vi "HFRR ADV v05 new software.vi"() -> ()   [LabVIEW 2025] (continued)
              tunnel: [w2074] -> w1919 mode=indexing
              tunnel: [w2070] -> w1894 mode=indexing
              tunnel: [w2066] -> w1875 mode=indexing
              tunnel: [w2061] -> w1833 mode=indexing
              (unwired) TRUE ("line mode (F)")
              n1812 = Read from Text File "Read File"(file (use dialog)=w2097, error in=w2096) -> (text=w2062:string)  [unwired: 2 in, 3 out]
              n1813 = local write "String 7"(w2062) -> ()
              n1814 = String Subset(string=w2062, offset (0)=85, length (rest)=9 ("length (rest)")) -> (substring=w2065:string)
              n1815 = String Subset(string=w2062, offset (0)=35, length (rest)=9 ("length (rest)")) -> (substring=w2087:string)
              n1816 = String Subset(string=w2062, offset (0)=55, length (rest)=9 ("length (rest)")) -> (substring=w2073:string)
              n1817 = String Subset(string=w2062, offset (0)=25, length (rest)=9 ("length (rest)")) -> (substring=w2067:string)
              n1818 = String Subset(string=w2062, offset (0)=45, length (rest)=9 ("length (rest)")) -> (substring=w2075:string)
              n1819 = String Subset(string=w2062, offset (0)=0, length (rest)=14 ("length (rest)")) -> (substring=w2090:string)
              n1820 = String Subset(string=w2062, offset (0)=15, length (rest)=9 ("length (rest)")) -> (substring=w2093:string)
              n1821 = String Subset(string=w2062, offset (0)=65, length (rest)=9 ("length (rest)")) -> (substring=w2079:string)
              n1822 = Fract/Exp String To Number(string=w2065) -> (number=w2061:dbl)  [unwired: 3 in, 1 out]
              n1823 = Fract/Exp String To Number(string=w2087) -> (number=w2085:dbl)  [unwired: 3 in, 1 out]
              n1824 = Fract/Exp String To Number(string=w2073) -> (number=w2070:dbl)  [unwired: 3 in, 1 out]
              n1825 = Fract/Exp String To Number(string=w2067) -> (number=w2066:dbl)  [unwired: 3 in, 1 out]
              n1826 = Fract/Exp String To Number(string=w2075) -> (number=w2074:dbl)  [unwired: 3 in, 1 out]
              n1827 = Fract/Exp String To Number(string=w2090) -> (number=w2086:dbl)  [unwired: 3 in, 1 out]
              n1828 = Fract/Exp String To Number(string=w2093) -> (number=w2084:dbl)  [unwired: 3 in, 1 out]
              n1829 = Fract/Exp String To Number(string=w2079) -> (number=w2082:dbl)  [unwired: 3 in, 1 out]
              n1830 = Add(x=w2082, y=0.0) -> (x+y=w2078:dbl)
            }
            n1831 = for {
              N: w1970 -> [_]
              tunnel: w1977 -> [w2025]
              tunnel: w1976 -> [w2024]
              tunnel: [w2014] -> w1930 mode=indexing
              tunnel: [w2013] -> w1923 mode=indexing
              tunnel: w1967 -> [_]
              tunnel: [w2002] -> w1928 mode=indexing
              tunnel: [w2007] -> w1925 mode=indexing
              tunnel: [w2003] -> w1915 mode=indexing
              tunnel: [w1998] -> w1890 mode=indexing
              tunnel: [w1994] -> w1871 mode=indexing
              tunnel: [w1989] -> w1831 mode=indexing
              (unwired) 1.0 ("x")
              (unwired) TRUE ("line mode (F)")
              n1832 = Read from Text File "Read File"(file (use dialog)=w2025, error in=w2024) -> (text=w1990:string)  [unwired: 2 in, 3 out]
              n1833 = local write "String 12"(w1990) -> ()
              n1834 = String Subset(string=w1990, offset (0)=85, length (rest)=9 ("length (rest)")) -> (substring=w1992:string)
              n1835 = String Subset(string=w1990, offset (0)=35, length (rest)=9 ("length (rest)")) -> (substring=w2015:string)
              n1836 = String Subset(string=w1990, offset (0)=55, length (rest)=9 ("length (rest)")) -> (substring=w2000:string)
              n1837 = String Subset(string=w1990, offset (0)=25, length (rest)=9 ("length (rest)")) -> (substring=w1996:string)
              n1838 = String Subset(string=w1990, offset (0)=45, length (rest)=9 ("length (rest)")) -> (substring=w2005:string)
              n1839 = String Subset(string=w1990, offset (0)=15, length (rest)=9 ("length (rest)")) -> (substring=w2021:string)
              n1840 = String Subset(string=w1990, offset (0)=0, length (rest)=14 ("length (rest)")) -> (substring=w2018:string)
              n1841 = String Subset(string=w1990, offset (0)=65, length (rest)=9 ("length (rest)")) -> (substring=w2008:string)
              n1842 = Fract/Exp String To Number(string=w1992) -> (number=w1989:dbl)  [unwired: 3 in, 1 out]
              n1843 = Fract/Exp String To Number(string=w2015) -> (number=w2013:dbl)  [unwired: 3 in, 1 out]
              n1844 = Fract/Exp String To Number(string=w2000) -> (number=w1998:dbl)  [unwired: 3 in, 1 out]
              n1845 = Fract/Exp String To Number(string=w1996) -> (number=w1994:dbl)  [unwired: 3 in, 1 out]
              n1846 = Fract/Exp String To Number(string=w2005) -> (number=w2003:dbl)  [unwired: 3 in, 1 out]
              n1847 = Fract/Exp String To Number(string=w2021) -> (number=w2002:dbl)  [unwired: 3 in, 1 out]
              n1848 = Fract/Exp String To Number(string=w2018) -> (number=w2014:dbl)  [unwired: 3 in, 1 out]
              n1849 = Fract/Exp String To Number(string=w2008) -> (number=w2011:dbl)  [unwired: 3 in, 1 out]
              n1850 = Add(x=w2011, y=0.0) -> (x+y=w2007:dbl)
            }
            n1851 = Delete From Array(array=w1873, index=0) -> (array with subset deleted=w1846:dbl[])  [unwired: 1 in, 1 out]
            n1852 = Delete From Array(array=w1936, index=0) -> (array with subset deleted=w1909:dbl[])  [unwired: 1 in, 1 out]
            n1853 = Delete From Array(array=w1916, index=0) -> (array with subset deleted=w1904:dbl[])  [unwired: 1 in, 1 out]
            n1854 = Delete From Array(array=w1934, index=0) -> (array with subset deleted=w1935:dbl[])  [unwired: 1 in, 1 out]
            n1855 = call-poly <vilib>:"Mean.vi"("X"=w1846) -> ("mean"=→"КОФ2 4":dbl)  [unwired: 1 out]
            n1856 = call-poly <vilib>:"Mean.vi"("X"=w1909) -> ("mean"=→"КОФ3":dbl)  [unwired: 1 out]
            n1857 = call-poly <vilib>:"Mean.vi"("X"=w1904) -> ("mean"=→"CP3":dbl)  [unwired: 1 out]
            n1858 = Delete From Array(array=w1898, index=0) -> (array with subset deleted=w1825:dbl[])  [unwired: 1 in, 1 out]
            n1859 = Delete From Array(array=w1837, index=0) -> (array with subset deleted=w1824:dbl[])  [unwired: 1 in, 1 out]
            n1860 = Delete From Array(array=w1877, index=0) -> (array with subset deleted=w1848:dbl[])  [unwired: 1 in, 1 out]
            n1861 = Delete From Array(array=w1955, index=0) -> (array with subset deleted=w1910:dbl[])  [unwired: 1 in, 1 out]
            n1862 = Delete From Array(array=w1921, index=0) -> (array with subset deleted=w1906:dbl[])  [unwired: 1 in, 1 out]
            "array w/ subset deleted" <- w1906
            n1863 = Delete From Array(array=w1952, index=0) -> (array with subset deleted=w1953:dbl[])  [unwired: 1 in, 1 out]
            n1864 = call-poly <vilib>:"Mean.vi"("X"=w1848) -> ("mean"=→"КОФ2 2":dbl)  [unwired: 1 out]
            n1865 = call-poly <vilib>:"Mean.vi"("X"=w1910) -> ("mean"=→"КОФ1":dbl)  [unwired: 1 out]
            n1866 = Bundle "Bundle"(w1825, w1824) -> (w1830:cluster{dbl[], dbl[]})  [unwired: 1 in]
            n1867 = Bundle "Bundle"(w1825, w1953) -> (w1817:cluster{dbl[], dbl[]})  [unwired: 1 in]
            n1868 = Delete From Array(array=w1832, index=0) -> (array with subset deleted=w1820:dbl[])  [unwired: 1 in, 1 out]
            n1869 = Delete From Array(array=w1833, index=0) -> (array with subset deleted=w1822:dbl[])  [unwired: 1 in, 1 out]
            n1870 = Delete From Array(array=w1943, index=0) -> (array with subset deleted=w1944:dbl[])  [unwired: 1 in, 1 out]
            n1871 = Delete From Array(array=w1831, index=0) -> (array with subset deleted=w1818:dbl[])  [unwired: 1 in, 1 out]
            n1872 = Delete From Array(array=w1925, index=0) -> (array with subset deleted=w1926:dbl[])  [unwired: 1 in, 1 out]
            n1873 = Delete From Array(array=w1950, index=0) -> (array with subset deleted=w1856:dbl[])  [unwired: 1 in, 1 out]
            n1874 = Delete From Array(array=w1896, index=0) -> (array with subset deleted=w1852:dbl[])  [unwired: 1 in, 1 out]
            n1875 = Delete From Array(array=w1932, index=0) -> (array with subset deleted=w1854:dbl[])  [unwired: 1 in, 1 out]
            n1876 = Delete From Array(array=w1892, index=0) -> (array with subset deleted=w1850:dbl[])  [unwired: 1 in, 1 out]
            n1877 = Delete From Array(array=w1941, index=0) -> (array with subset deleted=w1855:dbl[])  [unwired: 1 in, 1 out]
            n1878 = Delete From Array(array=w1894, index=0) -> (array with subset deleted=w1851:dbl[])  [unwired: 1 in, 1 out]
            n1879 = Delete From Array(array=w1875, index=0) -> (array with subset deleted=w1847:dbl[])  [unwired: 1 in, 1 out]
            n1880 = Delete From Array(array=w1919, index=0) -> (array with subset deleted=w1905:dbl[])  [unwired: 1 in, 1 out]
            n1881 = Delete From Array(array=w1946, index=0) -> (array with subset deleted=w1907:dbl[])  [unwired: 1 in, 1 out]
            n1882 = Delete From Array(array=w1923, index=0) -> (array with subset deleted=w1853:dbl[])  [unwired: 1 in, 1 out]
            n1883 = Delete From Array(array=w1890, index=0) -> (array with subset deleted=w1849:dbl[])  [unwired: 1 in, 1 out]
            n1884 = Delete From Array(array=w1871, index=0) -> (array with subset deleted=w1845:dbl[])  [unwired: 1 in, 1 out]
            n1885 = Delete From Array(array=w1915, index=0) -> (array with subset deleted=w1903:dbl[])  [unwired: 1 in, 1 out]
            n1886 = Delete From Array(array=w1928, index=0) -> (array with subset deleted=w1908:dbl[])  [unwired: 1 in, 1 out]
            n1887 = Delete From Array(array=w1938, index=0) -> (array with subset deleted=w1821:dbl[])  [unwired: 1 in, 1 out]
            n1888 = Delete From Array(array=w1948, index=0) -> (array with subset deleted=w1823:dbl[])  [unwired: 1 in, 1 out]
            n1889 = Delete From Array(array=w1930, index=0) -> (array with subset deleted=w1819:dbl[])  [unwired: 1 in, 1 out]
            n1890 = Bundle "Bundle"(w1825, w1856) -> (w1843:cluster{dbl[], dbl[]})  [unwired: 1 in]
            n1891 = Bundle "Bundle"(w1825, w1910) -> (w1844:cluster{dbl[], dbl[]})  [unwired: 1 in]
            n1892 = Bundle "Bundle"(w1856, w1852) -> (w1858:cluster{dbl[], dbl[]})  [unwired: 1 in]
            n1893 = Bundle "Bundle"(w1821, w1820) -> (w1828:cluster{dbl[], dbl[]})  [unwired: 1 in]
            n1894 = Bundle "Bundle"(w1854, w1850) -> (w1860:cluster{dbl[], dbl[]})  [unwired: 1 in]
            n1895 = Bundle "Bundle"(w1821, w1854) -> (w1964:cluster{dbl[], dbl[]})  [unwired: 1 in]
            n1896 = Bundle "Bundle"(w1821, w1850) -> (w1888:cluster{dbl[], dbl[]})  [unwired: 1 in]
            n1897 = Bundle "Bundle"(w1821, w1909) -> (w1974:cluster{dbl[], dbl[]})  [unwired: 1 in]
            n1898 = Bundle "Bundle"(w1821, w1904) -> (w1912:cluster{dbl[], dbl[]})  [unwired: 1 in]
            n1899 = Bundle "Bundle"(w1821, w1935) -> (w1959:cluster{dbl[], dbl[]})  [unwired: 1 in]
            n1900 = Bundle "Bundle"(w1855, w1851) -> (w1859:cluster{dbl[], dbl[]})  [unwired: 1 in]
            n1901 = Bundle "Bundle"(w1823, w1822) -> (w1829:cluster{dbl[], dbl[]})  [unwired: 1 in]
            n1902 = Bundle "Bundle"(w1823, w1855) -> (w1966:cluster{dbl[], dbl[]})  [unwired: 1 in]
            n1903 = Bundle "Bundle"(w1823, w1851) -> (w1889:cluster{dbl[], dbl[]})  [unwired: 1 in]
            n1904 = Bundle "Bundle"(w1823, w1905) -> (w1913:cluster{dbl[], dbl[]})  [unwired: 1 in]
            n1905 = Bundle "Bundle"(w1823, w1907) -> (w1975:cluster{dbl[], dbl[]})  [unwired: 1 in]
            n1906 = Bundle "Bundle"(w1823, w1944) -> (w1957:cluster{dbl[], dbl[]})  [unwired: 1 in]
            n1907 = Bundle "Bundle"(w1853, w1849) -> (w1861:cluster{dbl[], dbl[]})  [unwired: 1 in]
            n1908 = Bundle "Bundle"(w1819, w1818) -> (w1827:cluster{dbl[], dbl[]})  [unwired: 1 in]
            n1909 = Bundle "Bundle"(w1819, w1853) -> (w1965:cluster{dbl[], dbl[]})  [unwired: 1 in]
            n1910 = Bundle "Bundle"(w1819, w1849) -> (w1887:cluster{dbl[], dbl[]})  [unwired: 1 in]
            n1911 = Bundle "Bundle"(w1819, w1903) -> (w1911:cluster{dbl[], dbl[]})  [unwired: 1 in]
            n1912 = Bundle "Bundle"(w1819, w1908) -> (w1973:cluster{dbl[], dbl[]})  [unwired: 1 in]
            n1913 = Bundle "Bundle"(w1819, w1926) -> (w1958:cluster{dbl[], dbl[]})  [unwired: 1 in]
            n1914 = call-poly <vilib>:"Mean.vi"("X"=w1906) -> ("mean"=→"CP1":dbl)  [unwired: 1 out]
            n1915 = call-poly <vilib>:"Mean.vi"("X"=w1847) -> ("mean"=→"КОФ2 3":dbl)  [unwired: 1 out]
            n1916 = call-poly <vilib>:"Mean.vi"("X"=w1905) -> ("mean"=→"CP2":dbl)  [unwired: 1 out]
            n1917 = call-poly <vilib>:"Mean.vi"("X"=w1907) -> ("mean"=→"КОФ2":dbl)  [unwired: 1 out]
            n1918 = call-poly <vilib>:"Mean.vi"("X"=w1845) -> ("mean"=→"КОФ2 5":dbl)  [unwired: 1 out]
            n1919 = call-poly <vilib>:"Mean.vi"("X"=w1903) -> ("mean"=→"CP4":dbl)  [unwired: 1 out]
            n1920 = call-poly <vilib>:"Mean.vi"("X"=w1908) -> ("mean"=→"КОФ4":dbl)  [unwired: 1 out]
            n1921 = Bundle "Bundle"(w1825, w1852) -> (w1816:cluster{dbl[], dbl[]})  [unwired: 1 in]
            n1922 = Bundle "Bundle"(w1825, w1906) -> (w1839:cluster{dbl[], dbl[]})  [unwired: 1 in]
            n1923 = Build Array "Build Array"(w1816, w1839) -> (w1842:cluster{dbl[], dbl[]}[])
            "XY Graph 17" <- w1842
            n1924 = Build Array "Build Array"(w1830, w1829, w1828, w1827) -> (→"Frequency ( Hz )":cluster{dbl[], dbl[]}[])
            n1925 = Build Array "Build Array"(w1858, w1859, w1860, w1861) -> (→"Air Temp ( °C ) vs Humidity ( % RH )":cluster{dbl[], dbl[]}[])
            n1926 = Build Array "Build Array"(w1843, w1966, w1964, w1965) -> (→"Air Temperature  ( °C )":cluster{dbl[], dbl[]}[])
            n1927 = Build Array "Build Array"(w1816, w1889, w1888, w1887) -> (→"Humidity ( %RH )":cluster{dbl[], dbl[]}[])
            n1928 = Build Array "Build Array"(w1844, w1975, w1974, w1973) -> (→"Coefficient Of Friction":cluster{dbl[], dbl[]}[])
            n1929 = Build Array "Build Array"(w1839, w1913, w1912, w1911) -> (→"Sample Temperature ( °C )":cluster{dbl[], dbl[]}[])
            n1930 = Build Array "Build Array"(w1817, w1957, w1959, w1958) -> (→"XY Graph 13":cluster{dbl[], dbl[]}[])
            n1931 = Bundle "Bundle"(w1825, w1848) -> (w1870:cluster{dbl[], dbl[]})  [unwired: 1 in]
            n1932 = Bundle "Bundle"(w1821, w1846) -> (w1868:cluster{dbl[], dbl[]})  [unwired: 1 in]
            n1933 = Bundle "Bundle"(w1823, w1847) -> (w1869:cluster{dbl[], dbl[]})  [unwired: 1 in]
            n1934 = Bundle "Bundle"(w1819, w1845) -> (w1867:cluster{dbl[], dbl[]})  [unwired: 1 in]
            n1935 = Build Array "Build Array"(w1870, w1869, w1868, w1867) -> (→"Stroke ( mm )":cluster{dbl[], dbl[]}[])
            n1936 = local write "XY Graph 16"(w1842) -> ()
          }
          frame #2 {
          }
          frame #3 {
            n1937 = local write "Numeric 8"(0 ("Numeric 8")) -> ()
            n1938 = local write "Numeric 11"(0 ("Numeric 11")) -> ()
            n1939 = local write "Numeric 12"(0 ("Numeric 12")) -> ()
            n1940 = local write "Numeric 13"(0 ("Numeric 13")) -> ()
            n1941 = property on="OPEN" class="Bool (strict)"("Visible"=TRUE) -> ()  [unwired: 2 in, 2 out]
            n1942 = local read "String Control 2"() -> (w2142:string)
            n1943 = local read "String Control 4"() -> (w2141:string)
            n1944 = local read "String Control 6"() -> (w2140:string)
            n1945 = local read "String Control 8"() -> (w2139:string)
            n1946 = Match Pattern(string=w2142, regular expression="Samples / cycle :- ") -> (after substring=w2156:string)  [unwired: 1 in, 3 out]
            n1947 = Match Pattern(string=w2142, regular expression="Frequency :- ") -> (after substring=w2175:string)  [unwired: 1 in, 3 out]
            n1948 = Match Pattern(string=w2141, regular expression="Samples / cycle :- ") -> (after substring=w2152:string)  [unwired: 1 in, 3 out]
            n1949 = Match Pattern(string=w2141, regular expression="Frequency :- ") -> (after substring=w2170:string)  [unwired: 1 in, 3 out]
            n1950 = Match Pattern(string=w2140, regular expression="Samples / cycle :- ") -> (after substring=w2148:string)  [unwired: 1 in, 3 out]
            n1951 = Match Pattern(string=w2140, regular expression="Frequency :- ") -> (after substring=w2165:string)  [unwired: 1 in, 3 out]
            n1952 = Match Pattern(string=w2139, regular expression="Samples / cycle :- ") -> (after substring=w2144:string)  [unwired: 1 in, 3 out]
            n1953 = Match Pattern(string=w2139, regular expression="Frequency :- ") -> (after substring=w2160:string)  [unwired: 1 in, 3 out]
            n1954 = String Subset(string=w2156, length (rest)=6 ("length (rest)")) -> (substring=w2158:string)  [unwired: 1 in]
            n1955 = String Subset(string=w2175, length (rest)=9 ("length (rest)")) -> (substring=w2177:string)  [unwired: 1 in]
            n1956 = String Subset(string=w2152, length (rest)=6 ("length (rest)")) -> (substring=w2154:string)  [unwired: 1 in]
            n1957 = String Subset(string=w2170, length (rest)=9 ("length (rest)")) -> (substring=w2172:string)  [unwired: 1 in]
            n1958 = String Subset(string=w2148, length (rest)=6 ("length (rest)")) -> (substring=w2150:string)  [unwired: 1 in]
            n1959 = String Subset(string=w2165, length (rest)=9 ("length (rest)")) -> (substring=w2167:string)  [unwired: 1 in]
            n1960 = String Subset(string=w2144, length (rest)=6 ("length (rest)")) -> (substring=w2146:string)  [unwired: 1 in]
            n1961 = String Subset(string=w2160, length (rest)=9 ("length (rest)")) -> (substring=w2162:string)  [unwired: 1 in]
            n1962 = Fract/Exp String To Number(string=w2158) -> (number=w2138:dbl)  [unwired: 3 in, 1 out]
            n1963 = Fract/Exp String To Number(string=w2177) -> (number=w2178:dbl)  [unwired: 3 in, 1 out]
            n1964 = Fract/Exp String To Number(string=w2154) -> (number=w2137:dbl)  [unwired: 3 in, 1 out]
            n1965 = Fract/Exp String To Number(string=w2172) -> (number=w2173:dbl)  [unwired: 3 in, 1 out]
            n1966 = Fract/Exp String To Number(string=w2150) -> (number=w2136:dbl)  [unwired: 3 in, 1 out]
            n1967 = Fract/Exp String To Number(string=w2167) -> (number=w2168:dbl)  [unwired: 3 in, 1 out]
            n1968 = Fract/Exp String To Number(string=w2146) -> (number=w2135:dbl)  [unwired: 3 in, 1 out]
            n1969 = Fract/Exp String To Number(string=w2162) -> (number=w2163:dbl)  [unwired: 3 in, 1 out]
            n1970 = local write "sample1"(w2138) -> ()
            n1971 = local write "freq1"(w2178) -> ()
            n1972 = local write "sample2"(w2137) -> ()
            n1973 = local write "freq2"(w2173) -> ()
            n1974 = local write "sample3"(w2136) -> ()
            n1975 = local write "freq3"(w2168) -> ()
            n1976 = local write "sample4"(w2135) -> ()
            n1977 = local write "freq 4"(w2163) -> ()
          }
        }
      }
    }
    n1978 = case shown="True" w1627 {
      selector: w1627 -> [_ w1755]
      frame False {
      }
      frame True {
        n1979 = Not(x=w1755) -> (.not. x?=w1751:bool)
        n1980 = local write "service 3"(w1751) -> ()
        n1981 = local write "OPEN 6"(w1751) -> ()
        n1982 = call <vilib>:"System Exec.vi"("wait until completion? (T)"=TRUE, "command line"="C:\\LAB-IQ\\Scar View.exe") -> ("error out"=→"error out 5":errorcluster)  [unwired: 6 in, 3 out]
      }
    }
    n1983 = case shown="\"Acquire\", Default" w1638 {
      frame "Acquire", Default {
        w2651 = 0.2 ("y")
        w2656 = 1.0 ("y")
        w2657 = 0.8 ("y")
        # "Elapsed time\ncof\nstroke\nAir temp\nTemp\nHumidity"
        n1984 = disable-structure shown="Disabled" {
          frame Disabled {
            n1985 = local read "Flag"() -> (w2674:dbl)
            n1986 = local read "RUN"() -> (w2671:bool)
            n1987 = Not(x=w2671) -> (.not. x?=w2670:bool)
            n1988 = Equal?(x=w2674, y=10.0) -> (x = y?=w2672:bool)
            n1989 = And(x=w2672, y=w2670) -> (x .and. y?=w2669:bool)
            n1990 = case shown="True" w2669 {
              frame False {
              }
              frame True {
                w2675 = FALSE ("Heater Button")
                n1991 = local write "Humidity"(w2675) -> ()
                n1992 = local write "Heater Button"(w2675) -> ()
              }
            }
          }
          frame Enabled {
          }
        }
        n1993 = disable-structure shown="Disabled" {
          frame Disabled {
            n1994 = case shown="True" {
              selector: _ -> [_ _]
              frame False {
              }
              frame True {
                w2766 = TRUE ("Heater")
                n1995 = local write "Humidity"(w2766) -> ()
                n1996 = local write "Heater Button"(w2766) -> ()
                n1997 = local read "TEST STANDARD"() -> (w2769:T3)
                n1998 = local read "TEST STANDARD"() -> (w2764:T3)
                n1999 = Equal?(x=w2769, y=enum16{"ASTM D6079", "ISO 12156", "Custom"}."ISO 12156" ("Test Standard")) -> (x = y?=w2767:bool)
                n2000 = Equal?(x=w2764, y=enum16{"ASTM D6079", "ISO 12156", "Custom"}."ASTM D6079" ("Test Standard")) -> (x = y?=w2763:bool)
                n2001 = case shown="True" w2767 {
                  frame False {
                  }
                  frame True {
                    n2002 = local write "Heater"(TRUE ("Heater")) -> ()
                    n2003 = local write "airtempflg"(FALSE ("airtempflg")) -> ()
                  }
                }
                n2004 = case shown="True" w2763 {
                  frame False {
                  }
                  frame True {
                    n2005 = local write "Heater"(FALSE ("Heater")) -> ()
                    n2006 = local write "airtempflg"(TRUE ("airtempflg")) -> ()
                  }
                }
              }
            }
          }
          frame Enabled {
          }
        }
        n2007 = stacked-sequence {
          frame #0 {
            n2008 = case shown="True" "RST FF" {
              frame False {
              }
              frame True {
                w2832 = 0.0 ("X Scale.Range:Maximum")
                n2009 = property on="Frictional Force ( N )" class="WFChart (strict)"("XScale.Maximum"=600.0 ("X Scale.Range:Maximum"), "XScale.Minimum"=w2832, "YScale.Maximum"=10.0 ("Y Scale.Range:Maximum"), "YScale.Minimum"=w2832) -> ()  [unwired: 2 in, 2 out]
              }
            }
          }
          frame #1 {
            n2010 = case shown="True" "RST TEMP" {
              frame False {
              }
              frame True {
                n2011 = property on="Temperature ( Deg C )" class="WFChart (strict)"("XScale.Minimum"=0.0 ("X Scale.Range:Minimum"), "XScale.Maximum"=600.0 ("X Scale.Range:Maximum"), "YScale.Minimum"=0.0 ("Y Scale.Range:Minimum"), "YScale.Maximum"=100.0 ("Y Scale.Range:Maximum")) -> ()  [unwired: 2 in, 2 out]
              }
            }
          }
          frame #2 {
            n2012 = case shown="True" "RSTCOF" {
              frame False {
              }
              frame True {
                n2013 = property on="Coefficient of Friction" class="WFChart (strict)"("XScale.Minimum"=0.0 ("X Scale.Range:Minimum"), "XScale.Maximum"=600.0 ("X Scale.Range:Maximum"), "YScale.Maximum"=1.0 ("X Scale.Range:Minimum"), "YScale.Minimum"=0.0 ("X Scale.Range:Minimum")) -> ()  [unwired: 2 in, 2 out]
              }
            }
          }
          frame #3 {
            n2014 = case shown="True" "RSTCOF 2" {
              frame False {
              }
              frame True {
                (unwired) 100.0 ("Y Scale.Range:Maximum")
                (unwired) 0.0 ("Y Scale.Range:Minimum")
                (unwired) 600.0 ("X Scale.Range:Maximum")
                (unwired) 0.0 ("X Scale.Range:Minimum")
              }
            }
          }
          frame #4 {
            n2015 = case shown="True" "RSTCOF 3" {
              frame False {
              }
              frame True {
                n2016 = property on="Electrical Contact Resistance ( % )" class="WFChart (strict)"("XScale.Minimum"=0.0 ("X Scale.Range:Minimum"), "XScale.Maximum"=600.0 ("X Scale.Range:Maximum"), "YScale.Minimum"=0.0 ("Y Scale.Range:Minimum"), "YScale.Maximum"=100.0 ("Y Scale.Range:Maximum")) -> ()  [unwired: 2 in, 2 out]
              }
            }
          }
        }
        n2017 = disable-structure shown="Disabled" {
          frame Disabled {
            n2018 = case shown="True" {
              selector: _ -> [_ _]
              frame False {
              }
              frame True {
                n2019 = local read "zflag 2"() -> (w2733:dbl)
                n2020 = local read "yflag"() -> (w2735:dbl)
                n2021 = Equal?(x=w2735, y=2.0 ("tflag")) -> (x = y?=w2737:bool)
                n2022 = Equal?(x=w2733, y=3.0 ("tflag")) -> (x = y?=w2736:bool)
                n2023 = And(x=w2737, y=w2736) -> (x .and. y?=w2731:bool)
                n2024 = case shown="True" w2731 {
                  frame False {
                  }
                  frame True {
                    w2762 = 0.0 ("zflag")
                    n2025 = local write "zflag"(w2762) -> ()
                    n2026 = local write "zflag 2"(w2762) -> ()
                    n2027 = Delete(path (use dialog)=path "C:/LAB-IQ-NXT/WO 2449 TT.sig" ("file path (dialog if empty)")) -> (deleted path=w2761:path)  [unwired: 4 in, 2 out]
                    n2028 = Delete(path (use dialog)=path "C:/LAB-IQ-NXT/WO 2449 TRH.sig" ("file path (dialog if empty)")) -> (deleted path=w2756:path)  [unwired: 4 in, 2 out]
                    n2029 = local read "SEN.RUN HRS"() -> (w2748:dbl)
                    n2030 = local read "SENSOR TIME"() -> (w2746:dbl)
                    n2031 = call <vilib>:"compatOverwrite.vi"("overwrite (F)"=TRUE) -> ("overwrite?"=w2738:T23)
                    n2032 = call <vilib>:"compatOverwrite.vi"("overwrite (F)"=TRUE) -> ("overwrite?"=w2742:T23)
                    n2033 = local read "Total No. of Tests"() -> (w2749:dbl)
                    n2034 = Add(x=w2746, y=w2748) -> (x+y=w2747:dbl)
                    "SEN.RUN HRS" <- w2747
                    n2035 = Open/Create/Replace File(file path (use dialog)=w2761, operation (0:open)=w2738) -> (refnum out=w2739:refnum<file>, error out=w2740:errorcluster)  [unwired: 4 in, 1 out]
                    n2036 = Open/Create/Replace File(file path (use dialog)=w2756, operation (0:open)=w2742) -> (refnum out=w2743:refnum<file>, error out=w2744:errorcluster)  [unwired: 4 in, 1 out]
                    n2037 = Deny Access(4:w2740, 6:T21."deny none" ("deny mode (2)"), 7:w2739) -> (3:w2760:refnum<file>)  [unwired: 1 out]
                    n2038 = Deny Access(4:w2744, 6:T21."deny none" ("deny mode (2)"), 7:w2743) -> (3:w2752:refnum<file>)  [unwired: 1 out]
                    n2039 = Number To Decimal String(number=w2749) -> (decimal integer string=w2757:string)  [unwired: 1 in]
                    n2040 = Number To Decimal String(number=w2747) -> (decimal integer string=w2753:string)  [unwired: 1 in]
                    n2041 = Write to Binary File(file (use dialog)=w2760, data=w2757, 5:FALSE ("prepend array or string size? (T)")) -> ()  [unwired: 3 in, 3 out]
                    n2042 = Write to Binary File(file (use dialog)=w2752, data=w2753, 5:FALSE ("prepend array or string size? (T)")) -> ()  [unwired: 3 in, 3 out]
                  }
                }
              }
            }
          }
          frame Enabled {
          }
        }
        n2043 = local read "RUN"() -> (w2660:bool)
        n2044 = local read "run replace"() -> (w2664:bool)
        n2045 = local read "run replace"() -> (w2663:bool)
        n2046 = case shown="True" w2660 {
          frame False {
            n2047 = local write "run replace"(FALSE ("run replace")) -> ()
          }
          frame True {
            "run replace" <- TRUE ("run replace")
          }
        }
        n2048 = local read "RUN"() -> (w2668:bool)
        n2049 = local read "Set Temp"() -> (w2630:dbl)
        n2050 = local read "SetTemp"() -> (w2632:dbl)
        n2051 = case shown="False" w2668 {
          tunnel: [FALSE ("TEST RUNNING") TRUE ("TEST RUNNING")] -> w2667
          frame False {
            w2851 = 0.0 ("Flag")
            n2052 = local write "Elapsed time"(0.0 ("elapsedtime")) -> ()
            n2053 = local write "Time Remaining"(w2851) -> ()
            n2054 = local write "Flag"(w2851) -> ()
            n2055 = local write "Remaining Time"(w2851) -> ()
          }
          frame True {
            n2056 = local write "Flag"(10.0 ("Flag")) -> ()
          }
        }
        n2057 = case shown="False" w2664 {
          frame False {
            n2058 = local read "zflag"() -> (→"zflag 2":dbl)
            n2059 = local write "yflag"(2.0 ("tflag")) -> ()
            n2060 = local write "FLAG 4"(0.0 ("FLAG")) -> ()
          }
          frame True {
            n2061 = local write "yflag"(1.0 ("tflag")) -> ()
            n2062 = local write "zflag"(3.0 ("zflag")) -> ()
          }
        }
        n2063 = local read "acq 2"() -> (w2662:bool)
        n2064 = local read "AIR TEMP"() -> (w2625:dbl)
        n2065 = local read "Amb temp"() -> (w2629:dbl)
        n2066 = case shown="True" "Save & Continue" {
          frame False {
          }
          frame True {
            "acq 2" <- TRUE ("acq 2")
          }
        }
        n2067 = local read "Set Rh"() -> (w2631:dbl)
        n2068 = Add(x=w2632, y=w2657) -> (x+y=w2658:dbl)
        n2069 = Subtract(x=w2632, y=w2657) -> (x-y=w2659:dbl)
        n2070 = Add(x=w2630, y=w2651) -> (x+y=w2652:dbl)
        n2071 = Subtract(x=w2630, y=w2651) -> (x-y=w2653:dbl)
        n2072 = And(x=w2662, y=w2663) -> (x .and. y?=w2661:bool)
        n2073 = Greater Or Equal?(x=w2625, y=15.0) -> (x >= y?=w2626:bool)
        "powstat" <- w2626
        n2074 = local read "Humidity ( %RH )"() -> (w2628:dbl)
        n2075 = case shown="True" "Save & Continue" {
          frame False {
          }
          frame True {
            n2076 = while {
              tunnel: "0123456789abcdefghijklmnopqrstuvwxyzABCDEFGHIJKLMNOPQRSTUVWXYZ" ("string 2") -> [w2822]
              shift-right: [w2820] -> w2815
              shift-left: "" -> [w2819]
              i -> [w2829]
              stop <- w2828 stop-if-true
              n2077 = Random Number (0-1)() -> (number: 0 to 1=w2823:dbl)
              n2078 = Multiply(x=w2823, y=62.0) -> (x*y=w2825:dbl)
              n2079 = Decrement(x="Length") -> (x-1=w2818:i16)
              n2080 = To Word Integer(number=w2825) -> (16bit integer=w2826:i16)
              n2081 = String Subset(string=w2822, offset (0)=w2826, length (rest)=1 ("length (rest)")) -> (substring=w2821:string)
              n2082 = Greater Or Equal?(x=w2829, y=w2818) -> (x >= y?=w2828:bool)
              n2083 = Concatenate Strings(w2821, w2819) -> (w2820:string)
            }
            n2084 = local write "UUID"(w2815) -> ()
          }
        }
        n2085 = In Range and Coerce(upper limit=w2658, x=w2629, lower limit=w2659) -> (In Range?=w2648:bool)  [unwired: 1 out]
        n2086 = Add(x=w2631, y=w2656) -> (x+y=w2655:dbl)
        n2087 = Subtract(x=w2631, y=w2656) -> (x-y=w2654:dbl)
        n2088 = local read "TEMP"() -> (w2627:dbl)
        n2089 = case shown="True" "Save & Continue" {
          frame False {
          }
          frame True {
            n2090 = local read "Operator ID"() -> (w3136:string)
            n2091 = local read "FILE"() -> (w3142:string)
            n2092 = String Length(string=w3142) -> (length=w3140:i32)
            n2093 = String Length(string=w3136) -> (length=w3137:i32)
            n2094 = Greater?(x=w3140, y=0) -> (0:w3139:bool)
            n2095 = Greater?(x=w3137, y=0) -> (0:w3135:bool)
            n2096 = And(x=w3139, y=w3135) -> (x .and. y?=w3134:bool)
            n2097 = case shown="True" w3134 {
              frame False {
                n2098 = stacked-sequence {
                  frame #0 {
                    n2099 = One Button Dialog(message="Please Enter a File Name and Operator ID to save data !", button name ("OK")="Ok") -> ()  [unwired: 1 out]
                  }
                  frame #1 {
                    n2100 = local write "Save & Continue"(FALSE ("OK Button")) -> ()
                  }
                }
                n2101 = local write "Save & Continue"(FALSE ("OK Button")) -> ()
              }
              frame True {
                n2102 = stacked-sequence {
                  frame #0 {
                    n2103 = local read "FILE"() -> (w3148:string)
                    n2104 = call "file check.vi"("file name in"=w3148) -> ("file name out"=w3147:string)  [unwired: 9 in, 1 out]
                    n2105 = call <vilib>:"Application Directory.vi"() -> ("Application Directory"=w3158:path)
                    n2106 = Build Path(base path=w3158, name or relative path="data") -> (appended path=w3157:path)
                    n2107 = call <vilib>:"Trim Whitespace.vi"("string"=w3147) -> ("trimmed string"=w3155:string)  [unwired: 1 in]
                    n2108 = call <vilib>:"Trim Whitespace.vi"("string"=w3147) -> ("trimmed string"=w3156:string)  [unwired: 1 in]
                    n2109 = List Folder(path=w3157) -> (folder names=w3153:string[])  [unwired: 3 in, 3 out]
                    n2110 = Match Pattern(string=w3155, regular expression="_(") -> (before substring=w3152:string)  [unwired: 1 in, 3 out]
                    n2111 = for {
                      tunnel: w3153 -> [w3167] mode=indexing
                      tunnel: w3152 -> [w3165]
                      shift-right: [w3163] -> w3150
                      shift-left: bool[] [] -> [w3164]
                      n2112 = Match Pattern(string=w3167, regular expression="_(") -> (before substring=w3166:string)  [unwired: 1 in, 3 out]
                      n2113 = Equal?(x=w3166, y=w3165) -> (x = y?=w3162:bool)
                      n2114 = case shown="True" w3162 {
                        tunnel: w3162 -> [_ w3170]
                        tunnel: w3164 -> [w3169 w3172]
                        tunnel: [w3169 w3171] -> w3163
                        frame False {
                        }
                        frame True {
                          n2115 = Insert Into Array(array=w3172, new element=w3170) -> (w3171:bool[])  [unwired: 1 in]
                        }
                      }
                    }
                    n2116 = Equal?(x=w3153, y=w3152) -> (x = y?=w3161:bool[])
                    n2117 = Or Array Elements(Boolean array=w3161) -> (logical OR=w3160:bool)
                    n2118 = Array Size(array=w3150) -> (size(s)=w3149:i32)
                    n2119 = case shown="True" w3160 {
                      tunnel: w3156 -> [_ w3180]
                      tunnel: w3149 -> [_ w3173]
                      frame False {
                      }
                      frame True {
                        n2120 = Number To Decimal String(number=w3173) -> (decimal integer string=w3176:string)  [unwired: 1 in]
                        n2121 = Search/Split String(string=w3180, search string/char (-)="_(" ("regular expression")) -> (substring before match=w3178:string)  [unwired: 1 in, 2 out]
                        n2122 = Concatenate Strings(w3178, "_(" ("regular expression"), w3176, ")" ("regular expression")) -> (w3174:string)
                        n2123 = local write "FILE"(w3174) -> ()
                      }
                    }
                  }
                  frame #1 {
                    w3182 = 0.0
                    w3195 = cluster{"y":dbl, dbl, "y":dbl}[] [] ("History Data")
                    w3196 = FALSE ("Heater Button")
                    (unwired) ")!" ("string")
                    (unwired) ")" ("string")
                    w3194 = dbl[] [] ("History Data")
                    w3200 = "\r"
                    # "C:\\WinDucom\\Data\\"
                    # "C:\\LAB-IQ-NXT\\data"
                    n2124 = local write "Humidity ( %RH )"(w3182) -> ()
                    n2125 = local write "Frequency ( Hz )"(w3182) -> ()
                    n2126 = local write "Stroke 3"(w3182) -> ()
                    n2127 = local write "speedop"(0.0 ("PIDclk 2")) -> ()
                    n2128 = local write "Set Temp 2"(65.0 ("Set Temp 2")) -> ()
                    n2129 = local write "AIR TEMP"(w3182) -> ()
                    n2130 = local write "clk"(0.0 ("clk")) -> ()
                    n2131 = local write "Stroke 4"(w3182) -> ()
                    n2132 = local write "COF 2"(w3182) -> ()
                    n2133 = local write "TEMP"(w3182) -> ()
                    n2134 = local write "ecr 3"(w3182) -> ()
                    n2135 = local write "FF 3"(w3182) -> ()
                    n2136 = local write "FF 2"(w3182) -> ()
                    n2137 = property on="Humidity ( %RH )" class="WFChart (strict)"("History Data"=w3194) -> ()  [unwired: 2 in, 2 out]
                    n2138 = property on="Coefficient of Friction" class="WFChart (strict)"("History Data"=w3194) -> ()  [unwired: 2 in, 2 out]
                    n2139 = property on="Coefficient of Friction" class="WFChart (strict)"("History Data"=w3194) -> ()  [unwired: 2 in, 2 out]
                    n2140 = property on="Frictional Force ( N )" class="WFChart (strict)"("History Data"=w3194) -> ()  [unwired: 2 in, 2 out]
                    n2141 = property on="Electrical Contact Resistance ( % )" class="WFChart (strict)"("History Data"=w3194) -> ()  [unwired: 2 in, 2 out]
                    n2142 = property on="Electrical Contact Resistance ( % )" class="WFChart (strict)"("History Data"=w3194) -> ()  [unwired: 2 in, 2 out]
                    n2143 = property on="Temperature ( Deg C )" class="WFChart (strict)"("History Data"=w3194) -> ()  [unwired: 2 in, 2 out]
                    n2144 = property on="Frictional Force ( N )" class="WFChart (strict)"("History Data"=w3194) -> ()  [unwired: 2 in, 2 out]
                    n2145 = property on="Coefficient of Friction" class="WFChart (strict)"("History Data"=w3194) -> ()  [unwired: 2 in, 2 out]
                    n2146 = property on="Frictional Force ( N )" class="WFChart (strict)"("History Data"=w3194) -> ()  [unwired: 2 in, 2 out]
                    n2147 = property on="Electrical Contact Resistance ( % )" class="WFChart (strict)"("History Data"=w3194) -> ()  [unwired: 2 in, 2 out]
                    n2148 = property on="Temperature ( Deg C )" class="WFChart (strict)"("History Data"=w3194) -> ()  [unwired: 2 in, 2 out]
                    n2149 = property on="Humidity ( %RH )" class="WFChart (strict)"("History Data"=w3194) -> ()  [unwired: 2 in, 2 out]
                    n2150 = property on="Stroke ( mm )" class="WFChart (strict)"("History Data"=w3195) -> ()  [unwired: 2 in, 2 out]
                    n2151 = property on="Stroke ( mm )" class="WFChart (strict)"("History Data"=w3195) -> ()  [unwired: 2 in, 2 out]
                    n2152 = local write "Humidity"(w3196) -> ()
                    n2153 = local write "Heater Button"(w3196) -> ()
                    n2154 = local read "FILE"() -> (w3190:string)
                    n2155 = disable-structure shown="Enabled" {
                      disable-tunnel: [w3235 _] -> w3181
                      frame Enabled {
                        n2156 = local read "NORMAL LOAD"() -> (w3235:dbl)
                      }
                      frame Disabled {
                      }
                    }
                    n2157 = call "file check.vi"("file name in"=w3190) -> ("error out"=w3193:errorcluster, "file name out"=w3187:string)  [unwired: 9 in]
                    n2158 = call "FILE PATH CREATION.vi"("error in"=w3193, "FILE NAME :"=w3187) -> ("FILE OUT"=w3186:path)  [unwired: 8 in, 1 out]
                    n2159 = Concatenate Strings(w3187, ".dgf" ("Substring")) -> (w3192:string)
                    n2160 = Concatenate Strings(w3187, ".duf" ("Substring")) -> (w3188:string)
                    n2161 = Multiply(x=w3181, y=1.0) -> (x*y=w3214:dbl)
                    n2162 = Build Path(base path=w3186, name or relative path=w3192) -> (appended path=w3185:path)
                    n2163 = Build Path(base path=w3186, name or relative path=w3188) -> (appended path=w3184:path)
                    n2164 = Number To Fractional String(number=w3214, width (-)=i16 5, precision (6)=i16 2) -> (F-format string=w3222:string)  [unwired: 1 in]
                    n2165 = local read "Fuel Discription :"() -> (w3210:string)
                    n2166 = local read "Batch Ref Num :"() -> (w3198:string)
                    n2167 = Get Date/Time String(date format (0)=enum16{"short", "long", "abbreviated"}."short") -> (date string=w3233:string, time string=w3230:string)  [unwired: 2 in]
                    n2168 = local read "Remarks :"() -> (w3209:string)
                    n2169 = Concatenate Strings("Load :- " ("Substring"), w3222, " grams ," ("Substring")) -> (w3221:string)
                    n2170 = local read "String 41"() -> (w3201:string)
                    n2171 = Concatenate Strings(w3210) -> (w3211:string)
                    n2172 = Concatenate Strings(w3198) -> (w3197:string)
                    n2173 = Concatenate Strings("tested by") -> (w3205:string)
                    n2174 = Concatenate Strings("(" ("Substring"), w3233, ")" ("Substring"), w3230) -> (w3203:string)
                    "concatenated string" <- w3203
                    n2175 = Concatenate Strings(w3209, "," ("string")) -> (w3208:string)
                    n2176 = Concatenate Strings("  TIME;      COF;       STROKE;     AIR TEMP;  TEMP;  HUMIDITY;  ECR; PID-OUT; FREQUENCY" ("Substring"), "\r") -> (w3217:string)
                    n2177 = Concatenate Strings(w3201, w3200, "Fuel Discription :-" ("Substring"), w3211, w3200, w3221, w3200, "Batch Ref Num :-" ("Substring"), w3197, w3200, " Remarks :- " ("Substring"), w3208, w3200, " Date :- " ("Substring"), w3203, w3200, "Tested By :-" ("Substring"), w3205) -> (w3215:string)
                    "REMARKS" <- w3215
                    n2178 = call <vilib>:"Write Characters To File.vi"("append to file? (new file:F)"=FALSE, "character string"=w3217, "file path (dialog if empty)"=w3185) -> ()  [unwired: 2 in, 1 out]
                    n2179 = call <vilib>:"Write Characters To File.vi"("append to file? (new file:F)"=FALSE, "character string"=w3215, "file path (dialog if empty)"=w3184) -> ()  [unwired: 2 in, 1 out]
                  }
                  frame #2 {
                    n2180 = local write "Cycles elapsed"(0 ("Cycles elapsed")) -> ()
                    n2181 = local write "cyclecount"(0 ("cyclecount")) -> ()
                    n2182 = local write "Save & Continue"(FALSE ("OK")) -> ()
                    n2183 = local write "autostrtflg"(TRUE ("autostrtflg")) -> ()
                    n2184 = local write "Save"(FALSE ("Save")) -> ()
                    n2185 = Get Date/Time In Seconds() -> (seconds since 1Jan1904=w3240:timestamp)
                    n2186 = To Double Precision Float(number=w3240) -> (double precision float=w3239:dbl)
                    n2187 = local write "acq timer"(w3239) -> ()
                    n2188 = One Button Dialog(message="Please ensure sample is mounted properly and machine is ready in all aspects for testing !", button name ("OK")="Ok") -> ()  [unwired: 1 out]
                  }
                  frame #3 {
                    n2189 = stacked-sequence {
                      frame #0 {
                        n2190 = local write "Main Dashboard Buttons"(T1."Dashboard" ("Main Dashboard Buttons")) -> ()
                        n2191 = local write "Main Tab"(T2."Acquire" ("Main Tab")) -> ()
                      }
                      frame #1 {
                        n2192 = local write "EVENT LOG"("" ("EVENT LOG")) -> ()
                      }
                      frame #2 {
                        n2193 = Wait (ms)(milliseconds to wait=u32 50) -> ()  [unwired: 1 out]
                      }
                      frame #3 {
                        n2194 = disable-structure shown="Disabled" {
                          frame Disabled {
                            n2195 = local read "EVENT LOG"() -> (w3252:string)
                            n2196 = call "Event Log.vi"("Content"="Test Details", "EVENT LOG"=w3252) -> ("EVENT LOG"=w3251:string)  [unwired: 8 in, 1 out]
                            n2197 = local write "EVENT LOG"(w3251) -> ()
                          }
                          frame Enabled {
                          }
                        }
                      }
                      frame #4 {
                        n2198 = Wait (ms)(milliseconds to wait=u32 50) -> ()  [unwired: 1 out]
                      }
                      frame #5 {
                        n2199 = local read "FILE"() -> (w3254:string)
                        n2200 = Concatenate Strings("File Name :" ("Content"), w3254) -> (w3255:string)
                        n2201 = local read "EVENT LOG"() -> (w3258:string)
                        n2202 = call "Event Log.vi"("Content"=w3255, "EVENT LOG"=w3258) -> ("EVENT LOG"=w3257:string)  [unwired: 8 in, 1 out]
                        n2203 = local write "EVENT LOG"(w3257) -> ()
                      }
                      frame #6 {
                        n2204 = Wait (ms)(milliseconds to wait=u32 50) -> ()  [unwired: 1 out]
                      }
                      frame #7 {
                        n2205 = local read "Batch Ref Num :"() -> (w3260:string)
                        n2206 = Concatenate Strings("Batch Ref No :" ("Content"), w3260) -> (w3261:string)
                        n2207 = local read "EVENT LOG"() -> (w3264:string)
                        n2208 = call "Event Log.vi"("Content"=w3261, "EVENT LOG"=w3264) -> ("EVENT LOG"=w3263:string)  [unwired: 8 in, 1 out]
                        n2209 = local write "EVENT LOG"(w3263) -> ()
                      }
                      frame #8 {
                        n2210 = Wait (ms)(milliseconds to wait=u32 50) -> ()  [unwired: 1 out]
                      }
                      frame #9 {
                        n2211 = local read "tested by"() -> (w3266:string)
                        n2212 = Concatenate Strings("Tested By :" ("Content"), w3266) -> (w3267:string)
                        n2213 = local read "EVENT LOG"() -> (w3270:string)
                        n2214 = call "Event Log.vi"("Content"=w3267, "EVENT LOG"=w3270) -> ("EVENT LOG"=w3269:string)  [unwired: 8 in, 1 out]
                        n2215 = local write "EVENT LOG"(w3269) -> ()
                      }
                      frame #10 {
                        n2216 = Wait (ms)(milliseconds to wait=u32 50) -> ()  [unwired: 1 out]
                      }
                      frame #11 {
                        n2217 = local read "TEST STANDARD"() -> (w3273:T3)
                        n2218 = case shown="\"ASTM D6079\", Default" w3273 {
                          tunnel: ["ASTM D6079" "ISO 12156" "CEC F-096-A-06" "Custom"] -> w3272
                          frame "ASTM D6079", Default {
                          }
                          frame "ISO 12156" {
                          }
                          frame "CEC F-096-A-06" {
                          }
                          frame "Custom" {
                          }
                        }
                        n2219 = Concatenate Strings("Test Standard :" ("Content"), w3272) -> (w3274:string)
                        n2220 = local read "EVENT LOG"() -> (w3277:string)
                        n2221 = call "Event Log.vi"("Content"=w3274, "EVENT LOG"=w3277) -> ("EVENT LOG"=w3276:string)  [unwired: 8 in, 1 out]
                        n2222 = local write "EVENT LOG"(w3276) -> ()
                      }
                      frame #12 {
                        n2223 = Wait (ms)(milliseconds to wait=u32 50) -> ()  [unwired: 1 out]
                      }
                      frame #13 {
                        n2224 = local read "Fuel Discription :"() -> (w3283:string)
                        n2225 = Concatenate Strings("Fuel Description :" ("Content"), w3283) -> (w3284:string)
                        n2226 = local read "EVENT LOG"() -> (w3287:string)
                        n2227 = call "Event Log.vi"("Content"=w3284, "EVENT LOG"=w3287) -> ("EVENT LOG"=w3286:string)  [unwired: 8 in, 1 out]
                        n2228 = local write "EVENT LOG"(w3286) -> ()
                      }
                      frame #14 {
                        n2229 = Wait (ms)(milliseconds to wait=u32 50) -> ()  [unwired: 1 out]
                      }
                      frame #15 {
                        n2230 = local read "Remarks :"() -> (w3289:string)
                        n2231 = Concatenate Strings("Remarks :" ("Content"), w3289) -> (w3290:string)
                        n2232 = local read "EVENT LOG"() -> (w3293:string)
                        n2233 = call "Event Log.vi"("Content"=w3290, "EVENT LOG"=w3293) -> ("EVENT LOG"=w3292:string)  [unwired: 8 in, 1 out]
                        n2234 = local write "EVENT LOG"(w3292) -> ()
                      }
                      frame #16 {
                        n2235 = Wait (ms)(milliseconds to wait=u32 50) -> ()  [unwired: 1 out]
                      }
                      frame #17 {
                        n2236 = local read "Operator ID"() -> (w3295:string)
                        n2237 = Concatenate Strings("Operator ID :" ("Content"), w3295) -> (w3297:string)
                        n2238 = local read "EVENT LOG"() -> (w3299:string)
                        n2239 = call "Event Log.vi"("Content"=w3297, "EVENT LOG"=w3299) -> ("EVENT LOG"=w3298:string)  [unwired: 8 in, 1 out]
                        n2240 = local write "EVENT LOG"(w3298) -> ()
                      }
                      frame #18 {
                        n2241 = Wait (ms)(milliseconds to wait=u32 50) -> ()  [unwired: 1 out]
                      }
                      frame #19 {
                        n2242 = disable-structure shown="Disabled" {
                          frame Disabled {
                            n2243 = local read "EVENT LOG"() -> (w3303:string)
                            n2244 = call "Event Log.vi"("Content"="Test Parameter", "EVENT LOG"=w3303) -> ("EVENT LOG"=w3302:string)  [unwired: 8 in, 1 out]
                            n2245 = local write "EVENT LOG"(w3302) -> ()
                          }
                          frame Enabled {
                          }
                        }
                      }
                      frame #20 {
                        n2246 = Wait (ms)(milliseconds to wait=u32 50) -> ()  [unwired: 1 out]
                      }
                      frame #21 {
                        n2247 = local read "Set Hz"() -> (w3307:dbl)
                        n2248 = Number To Fractional String(number=w3307, precision (6)=i16 2) -> (F-format string=w3306:string)  [unwired: 2 in]
                        n2249 = Concatenate Strings("Set Frequency [Hz] :" ("Content"), w3306) -> (w3309:string)
                        n2250 = local read "EVENT LOG"() -> (w3311:string)
                        n2251 = call "Event Log.vi"("Content"=w3309, "EVENT LOG"=w3311) -> ("EVENT LOG"=w3310:string)  [unwired: 8 in, 1 out]
                        n2252 = local write "EVENT LOG"(w3310) -> ()
                      }
                      frame #22 {
                        n2253 = Wait (ms)(milliseconds to wait=u32 50) -> ()  [unwired: 1 out]
                      }
                      frame #23 {
                        n2254 = local read "NORMAL LOAD"() -> (w3314:dbl)
                        n2255 = Number To Fractional String(number=w3314, precision (6)=i16 2) -> (F-format string=w3315:string)  [unwired: 2 in]
                        n2256 = Concatenate Strings("Applied Load [grams] :" ("Content"), w3315) -> (w3317:string)
                        n2257 = local read "EVENT LOG"() -> (w3319:string)
                        n2258 = call "Event Log.vi"("Content"=w3317, "EVENT LOG"=w3319) -> ("EVENT LOG"=w3318:string)  [unwired: 8 in, 1 out]
                        n2259 = local write "EVENT LOG"(w3318) -> ()
                      }
                      frame #24 {
                        n2260 = Wait (ms)(milliseconds to wait=u32 50) -> ()  [unwired: 1 out]
                      }
                      frame #25 {
                        n2261 = local read "Set Strk"() -> (w3322:dbl)
                        n2262 = Number To Fractional String(number=w3322, precision (6)=i16 2) -> (F-format string=w3323:string)  [unwired: 2 in]
                        n2263 = Concatenate Strings("Set Stroke [mm] :" ("Content"), w3323) -> (w3325:string)
                        n2264 = local read "EVENT LOG"() -> (w3327:string)
                        n2265 = call "Event Log.vi"("Content"=w3325, "EVENT LOG"=w3327) -> ("EVENT LOG"=w3326:string)  [unwired: 8 in, 1 out]
                        n2266 = local write "EVENT LOG"(w3326) -> ()
                      }
                      frame #26 {
                        n2267 = Wait (ms)(milliseconds to wait=u32 50) -> ()  [unwired: 1 out]
                      }
                      frame #27 {
                        n2268 = local read "Set Temp"() -> (w3330:dbl)
                        n2269 = Number To Fractional String(number=w3330, precision (6)=i16 2) -> (F-format string=w3331:string)  [unwired: 2 in]
                        n2270 = Concatenate Strings("Set Temperature [deg C] :" ("Content"), w3331) -> (w3333:string)
                        n2271 = local read "EVENT LOG"() -> (w3335:string)
                        n2272 = call "Event Log.vi"("Content"=w3333, "EVENT LOG"=w3335) -> ("EVENT LOG"=w3334:string)  [unwired: 8 in, 1 out]
                        n2273 = local write "EVENT LOG"(w3334) -> ()
                      }
                      frame #28 {
                        n2274 = Wait (ms)(milliseconds to wait=u32 50) -> ()  [unwired: 1 out]
                      }
                      frame #29 {
                        n2275 = local read "Set Rh"() -> (w3338:dbl)
                        n2276 = Number To Fractional String(number=w3338, precision (6)=i16 2) -> (F-format string=w3339:string)  [unwired: 2 in]
                        n2277 = Concatenate Strings("Set Humidity [%RH] :" ("Content"), w3339) -> (w3341:string)
                        n2278 = local read "EVENT LOG"() -> (w3343:string)
                        n2279 = call "Event Log.vi"("Content"=w3341, "EVENT LOG"=w3343) -> ("EVENT LOG"=w3342:string)  [unwired: 8 in, 1 out]
                        n2280 = local write "EVENT LOG"(w3342) -> ()
                      }
                      frame #30 {
                        n2281 = Wait (ms)(milliseconds to wait=u32 50) -> ()  [unwired: 1 out]
                      }
                      frame #31 {
                        n2282 = local read "test time"() -> (w3346:dbl)
                        n2283 = Number To Fractional String(number=w3346, precision (6)=i16 1) -> (F-format string=w3347:string)  [unwired: 2 in]
                        n2284 = Concatenate Strings("Test Duration [mins] :" ("Content"), w3347) -> (w3349:string)
                        n2285 = local read "EVENT LOG"() -> (w3351:string)
                        n2286 = call "Event Log.vi"("Content"=w3349, "EVENT LOG"=w3351) -> ("EVENT LOG"=w3350:string)  [unwired: 8 in, 1 out]
                        n2287 = local write "EVENT LOG"(w3350) -> ()
                      }
                      frame #32 {
                        w3352 = dbl[] [] ("History Data")
                        w3353 = cluster{"y":dbl, dbl, "y":dbl}[] [] ("History Data")
                        w3354 = FALSE ("Visible")
                        n2288 = property on="Stroke ( mm )" class="WFChart (strict)"("History Data"=w3353) -> ()  [unwired: 2 in, 2 out]
